vi "Gx Trigger Detector Config.vi"(0 "Slot":i16=1, 5 "Slope":enum16{"Rising Edge", "Falling Edge"}(ring), 7 "Trigger Voltage":dbl format="%.2f", 11 "error in (no error)":errorcluster) -> (4 "Handle Out":i16, 15 "error out":errorcluster)   [LabVIEW 2010]
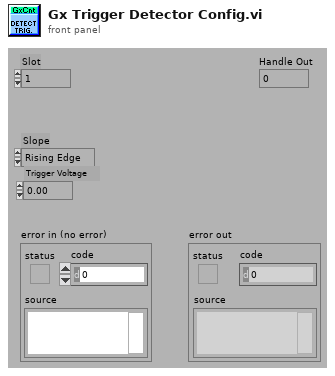
[diagram p1: front panel]
types:
  T1 = enum16{"Trigger Level Fixed", "Trigger Level Auto", "Trigger Level Hold Last"}
  T2 = enum16{"Filter Off", "Filter Auto", "Filter Value Fixed"}
  T3 = enum16{"Arm External", "Arm Off", "Arm Alternate"}
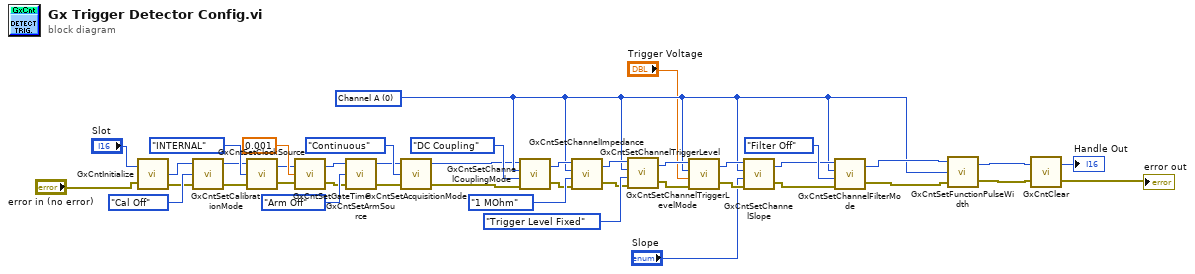
[diagram p0: block diagram]
diagram:
  w7 = i16 0 items=["Channel A", "Channel B"] ("Channel")
  n1 = call "GxCntInitialize.vi"("Slot"="Slot", "error in (no error)"="error in (no error)") -> ("Handle"=w25:i16, "error out"=w26:errorcluster)  [unwired: 1 out]
  n2 = call "GxCntSetCalibrationMode.vi"("error in (no error)"=w26, "Mode"=enum16{"Cal Off", "Cal Continuous", "Cal Once"}."Cal Off", "Handle"=w25) -> ("error out"=w23:errorcluster, "Handle copy"=w24:i16)
  n3 = call "GxCntSetClockSource.vi"("error in (no error)"=w23, "Source"=enum16{"INTERNAL", "EXTERNAL", "ALTERNATE"}."INTERNAL", "Handle"=w24) -> ("error out"=w38:errorcluster, "Handle copy"=w37:i16)
  n4 = call "GxCntSetGateTime.vi"("error in (no error)"=w38, "Seconds"=0.001, "Handle"=w37) -> ("error out"=w27:errorcluster, "Handle copy"=w28:i16)
  n5 = call "GxCntSetArmSource.vi"("error in (no error)"=w27, "Source"=T3."Arm Off", "Handle"=w28) -> ("error out"=w21:errorcluster, "Handle copy"=w22:i16)
  n6 = call "GxCntSetAcquisitionMode.vi"("error in (no error)"=w21, "Mode"=enum16{"Continuous", "Single", "Paced"}."Continuous", "Handle"=w22) -> ("error out"=w1:errorcluster, "Handle copy"=w2:i16)
  n7 = call "GxCntSetChannelCouplingMode.vi"("error in (no error)"=w1, "Mode"=enum16{"AC Coupling", "DC Coupling"}."DC Coupling", "Channel"=w7, "Handle"=w2) -> ("error out"=w20:errorcluster, "Handle copy"=w19:i16)
  n8 = call "GxCntSetChannelImpedance.vi"("error in (no error)"=w20, "Mode"=enum16{"1 MOhm", "50 Ohm"}."1 MOhm", "Channel"=w7, "Handle"=w19) -> ("error out"=w10:errorcluster, "Handle copy"=w11:i16)
  n9 = call "GxCntSetChannelTriggerLevelMode.vi"("error in (no error)"=w10, "Mode"=T1."Trigger Level Fixed", "Channel"=w7, "Handle"=w11) -> ("error out"=w8:errorcluster, "Handle copy"=w9:i16)
  n10 = call "GxCntSetChannelTriggerLevel.vi"("error in (no error)"=w8, "Voltage"="Trigger Voltage", "Channel"=w7, "Handle"=w9) -> ("error out"=w18:errorcluster, "Handle copy"=w17:i16)
  n11 = call "GxCntSetChannelSlope.vi"("error in (no error)"=w18, "Slope"="Slope", "Channel"=w7, "Handle"=w17) -> ("error out"=w15:errorcluster, "Handle copy"=w16:i16)
  n12 = call "GxCntSetChannelFilterMode.vi"("error in (no error)"=w15, "Mode"=T2."Filter Off", "Channel"=w7, "Handle"=w16) -> ("error out"=w13:errorcluster, "Handle copy"=w14:i16)
  n13 = call "GxCntSetFunctionPulseWidth.vi"("error in (no error)"=w13, "Channel"=w7, "Handle"=w14) -> ("error out"=w35:errorcluster, "Handle copy"=w36:i16)
  n14 = call "GxCntClear.vi"("error in (no error)"=w35, "Handle"=w36) -> ("error out"=→"error out":errorcluster, "Handle Out"=→"Handle Out":i16)
